vi "robot_server.vi"(11 "robot load":bool) -> ()   [LabVIEW 2020]
uses:
  status/stop software.vi
  status/emergency stop.vi
  status/robot pause.vi
  subvi/Robot-HL/small_scara_interface/small_scara_interface.lvlib
panel:
  out "count?":bool
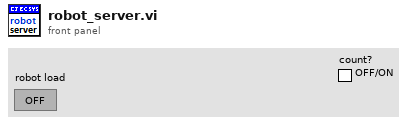
[diagram p1: front panel]
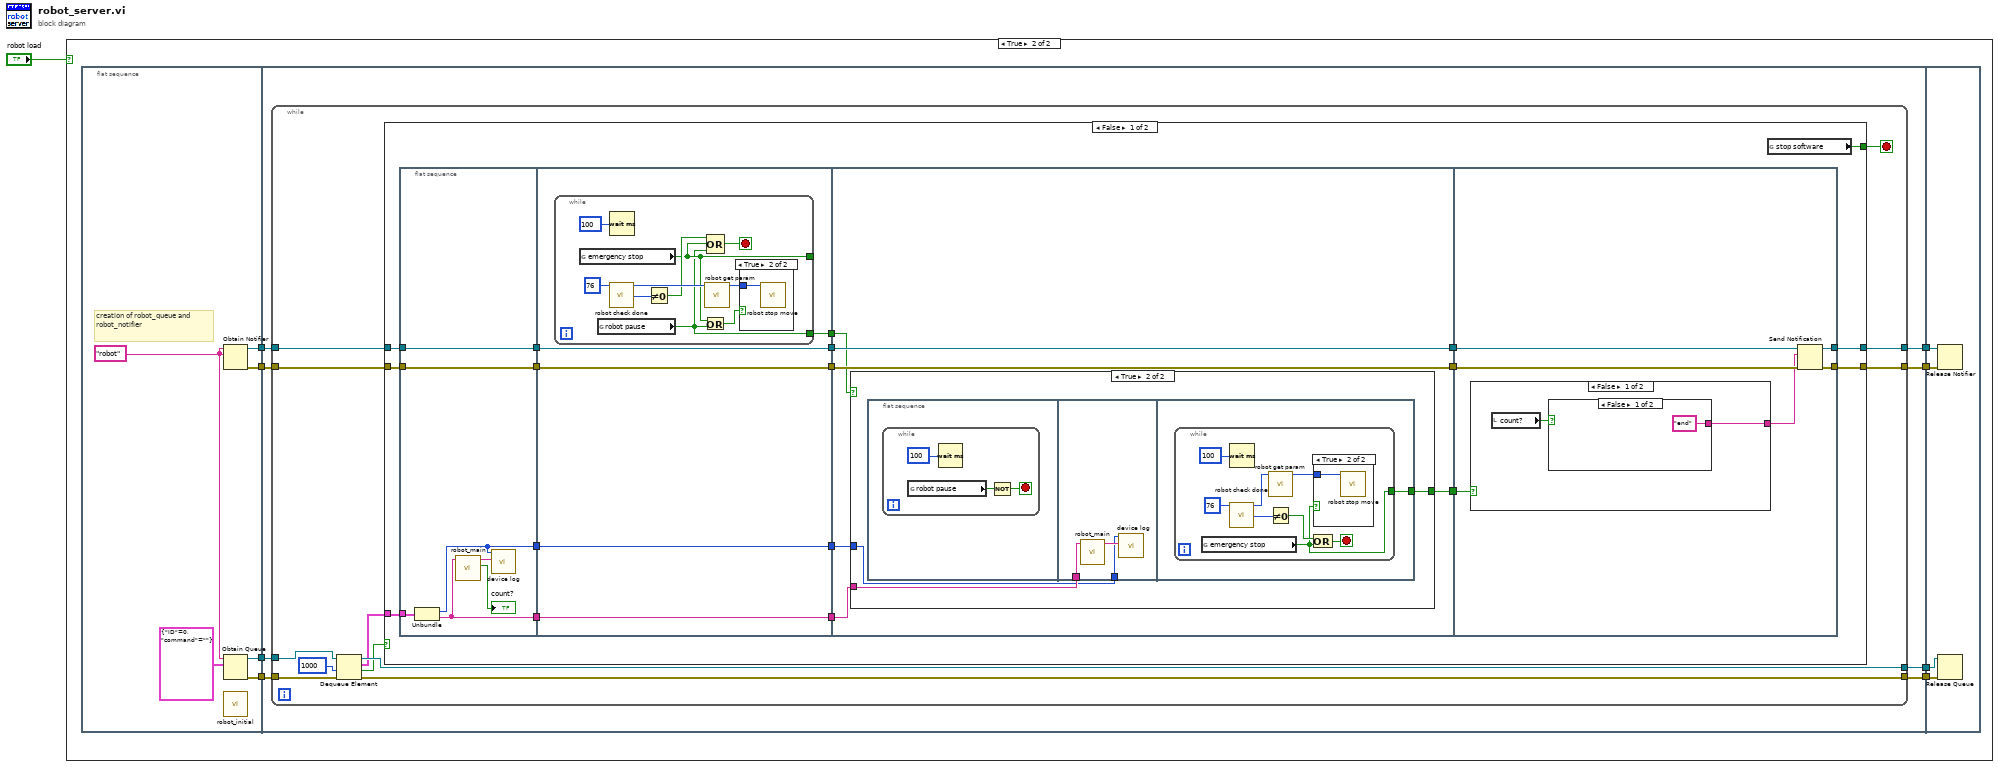
[diagram p0: block diagram]
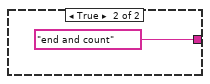
[diagram p6: hidden frame]
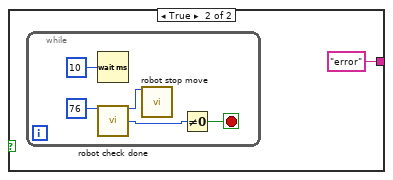
[diagram p7: hidden frame]
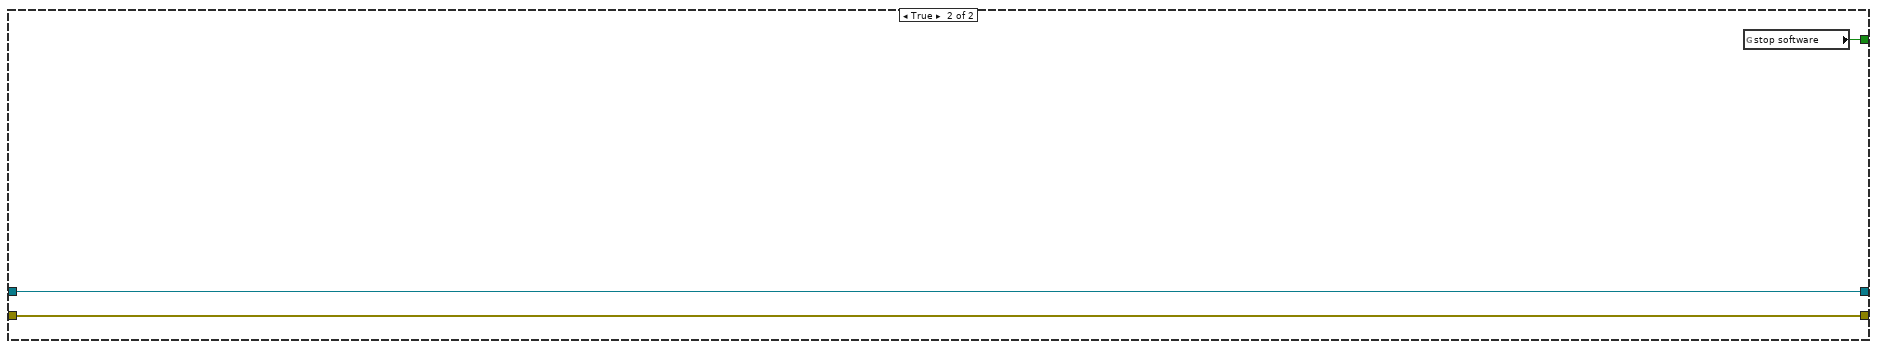
[diagram p8: hidden frame]
diagram:
  n1 = case shown="True" "robot load" {
    frame False {
    }
    frame True {
      n2 = flat-sequence {
        tunnel: [w15] -> w9
        tunnel: [w14] -> w8
        tunnel: [w13] -> w7
        tunnel: [w12] -> w6
        tunnel: w9 -> [w23]
        tunnel: w8 -> [w22]
        tunnel: w7 -> [w21]
        tunnel: w6 -> [w20]
        tunnel: [w19] -> w5
        tunnel: [w18] -> w4
        tunnel: [w17] -> w3
        tunnel: [w16] -> w2
        tunnel: w5 -> [w124]
        tunnel: w4 -> [w123]
        tunnel: w3 -> [w122]
        tunnel: w2 -> [w121]
        frame #0 {
          w11 = "robot" ("name (unnamed)")
          # "creation of robot_queue and robot_notifier"
          n3 = Obtain Notifier(name (unnamed)=w11, notification data type=w11) -> (notifier out=w13:refnum<notifier>, error out=w12:errorcluster)  [unwired: 2 in, 1 out]
          n4 = Obtain Queue(name (unnamed)=w11, element data type=cluster{"ID":i32, "command":string} {"ID"=0, "command"=""} ("参数")) -> (queue out=w15:refnum<queue>, error out=w14:errorcluster)  [unwired: 3 in, 1 out]
          n5 = call "robot_initial.vi"() -> ()  [unwired: 12 in]
        }
        frame #1 {
          n6 = while {
            tunnel: w23 -> [w34]
            tunnel: w22 -> [w33]
            tunnel: w21 -> [w31]
            tunnel: w20 -> [w30]
            tunnel: [w29] -> w19
            tunnel: [w28] -> w18
            tunnel: [w27] -> w17
            tunnel: [w26] -> w16
            stop <- w32 stop-if-true
            n7 = Dequeue Element(queue=w34, timeout in ms (-1)=1000, error in (no error)=w33) -> (queue out=w27:refnum<queue>, element=w25:cluster{"ID":i32, "command":string}, timed out?=w24:bool, error out=w26:errorcluster)
            n8 = case shown="False" w24 {
              tunnel: [w49 w118] -> w32
              tunnel: w31 -> [w53 w119]
              tunnel: w30 -> [w52 w120]
              tunnel: [w51 w119] -> w29
              tunnel: [w50 w120] -> w28
              tunnel: w25 -> [w48 _]
              frame False {
                n9 = flat-sequence {
                  tunnel: w53 -> [w60]
                  tunnel: [w60] -> w47
                  tunnel: w52 -> [w59]
                  tunnel: [w59] -> w46
                  tunnel: w48 -> [w58]
                  tunnel: [w55] -> w40
                  tunnel: [w54] -> w38
                  tunnel: w47 -> [w65]
                  tunnel: [w65] -> w45
                  tunnel: w46 -> [w64]
                  tunnel: [w64] -> w43
                  tunnel: [w63] -> w41
                  tunnel: w40 -> [w62]
                  tunnel: [w62] -> w39
                  tunnel: w38 -> [w61]
                  tunnel: [w61] -> w37
                  tunnel: w45 -> [w82]
                  tunnel: [w82] -> w44
                  tunnel: w43 -> [w81]
                  tunnel: [w81] -> w42
                  tunnel: w41 -> [w80]
                  tunnel: w39 -> [w79]
                  tunnel: w37 -> [w78]
                  tunnel: [w77] -> w36
                  tunnel: w44 -> [w107]
                  tunnel: w42 -> [w106]
                  tunnel: [w105] -> w51
                  tunnel: [w104] -> w50
                  tunnel: w36 -> [w102]
                  frame #0 {
                    n10 = Unbundle(w58) -> ("ID"=w54:i32, "command"=w55:string)
                    n11 = call "robot_main.vi"("input string"=w55) -> ("count?"=→"count?":bool, "output string"=w56:string)  [unwired: 9 in]
                    n12 = call "device log.vi"("new element/subarray"=w56, "worker ID"=w54) -> ()  [unwired: 10 in]
                  }
                  frame #1 {
                    n13 = while {
                      tunnel: [w67] -> _
                      tunnel: [w66] -> w63
                      stop <- w69 stop-if-true
                      n14 = global read "emergency stop.vi" "emergency stop"() -> (w67:bool)
                      n15 = global read "robot pause.vi" "robot pause"() -> (w66:bool)
                      n16 = call "robot check done.vi"("robot_id"=76) -> ("robot_id out"=w72:i32, "function return"=w73:i32)  [unwired: 12 in, 1 out]
                      n17 = Wait (ms)(milliseconds to wait=u32 100 ("等待时间（毫秒）")) -> ()  [unwired: 1 out]
                      n18 = Not Equal To 0?(x=w73) -> (x != 0?=w70:bool)
                      n19 = Or(x=w67, y=w66) -> (x .or. y?=w68:bool)
                      n20 = call "robot get param.vi"("robot_id"=w72) -> ("robot_id out"=w71:i32)  [unwired: 11 in, 3 out]
                      n21 = Compound Arithmetic op=OR(w70, w67, w66) -> (w69:bool)
                      n22 = case shown="True" w68 {
                        tunnel: w71 -> [_ w76]
                        frame False {
                        }
                        frame True {
                          n23 = call "robot stop move.vi"("robot_id"=w76) -> ()  [unwired: 12 in, 3 out]
                        }
                      }
                    }
                  }
                  frame #2 {
                    n24 = case shown="True" w80 {
                      tunnel: w79 -> [_ w85]
                      tunnel: w78 -> [_ w84]
                      tunnel: [_ w83] -> w77
                      frame False {
                      }
                      frame True {
                        n25 = flat-sequence {
                          tunnel: w85 -> [w90]
                          tunnel: w84 -> [w89]
                          tunnel: [w92] -> w83
                          frame #0 {
                            n26 = while {
                              stop <- w88 stop-if-true
                              n27 = global read "robot pause.vi" "robot pause"() -> (w87:bool)
                              n28 = Wait (ms)(milliseconds to wait=u32 100) -> ()  [unwired: 1 out]
                              n29 = Not(x=w87) -> (.not. x?=w88:bool)
                            }
                          }
                          frame #1 {
                            n30 = call "robot_main.vi"("input string"=w90) -> ("output string"=w91:string)  [unwired: 9 in, 1 out]
                            n31 = call "device log.vi"("new element/subarray"=w91, "worker ID"=w89) -> ()  [unwired: 10 in]
                          }
                          frame #2 {
                            n32 = while {
                              tunnel: [w94] -> w92
                              stop <- w93 stop-if-true
                              n33 = global read "emergency stop.vi" "emergency stop"() -> (w94:bool)
                              n34 = call "robot check done.vi"("robot_id"=76) -> ("robot_id out"=w97:i32, "function return"=w98:i32)  [unwired: 12 in, 1 out]
                              n35 = Wait (ms)(milliseconds to wait=u32 100 ("等待时间（毫秒）")) -> ()  [unwired: 1 out]
                              n36 = call "robot get param.vi"("robot_id"=w97) -> ("robot_id out"=w96:i32)  [unwired: 11 in, 3 out]
                              n37 = Not Equal To 0?(x=w98) -> (x != 0?=w95:bool)
                              n38 = case shown="True" w94 {
                                tunnel: w96 -> [_ w101]
                                frame False {
                                }
                                frame True {
                                n39 = call "robot stop move.vi"("robot_id"=w101) -> ()  [unwired: 12 in, 3 out]
                                }
                              }
                              n40 = Compound Arithmetic op=OR(w95, w94) -> (w93:bool)
                            }
                          }
                        }
                      }
                    }
                  }
                  frame #3 {
                    n41 = case shown="False" w102 {
                      tunnel: [w108 "error" ("notification")] -> w103
                      frame False {
                        n42 = local read "count?"() -> (w109:bool)
                        n43 = case shown="False" w109 {
                          tunnel: ["end" ("notification") "end and count" ("notification")] -> w108
                          frame False {
                          }
                          frame True {
                          }
                        }
                      }
                      frame True {
                        n44 = while {
                          stop <- w116 stop-if-true
                          n45 = Wait (ms)(milliseconds to wait=u32 10 ("等待时间（毫秒）")) -> ()  [unwired: 1 out]
                          n46 = call "robot check done.vi"("robot_id"=76) -> ("robot_id out"=w114:i32, "function return"=w113:i32)  [unwired: 12 in, 1 out]
                          n47 = call "robot stop move.vi"("robot_id"=w114) -> ()  [unwired: 12 in, 3 out]
                          n48 = Not Equal To 0?(x=w113) -> (x != 0?=w116:bool)
                        }
                      }
                    }
                    n49 = Send Notification(notification=w103, notifier=w107, error in (no error)=w106) -> (notifier out=w105:refnum<notifier>, error out=w104:errorcluster)
                  }
                }
                n50 = global read "stop software.vi" "stop software"() -> (w49:bool)
              }
              frame True {
                n51 = global read "stop software.vi" "stop software"() -> (w118:bool)
              }
            }
          }
        }
        frame #2 {
          n52 = Release Notifier(notifier=w124, error in (no error)=w123) -> ()  [unwired: 1 in, 3 out]
          n53 = Release Queue(queue=w122, error in (no error)=w121) -> ()  [unwired: 1 in, 3 out]
        }
      }
    }
  }
